vi "FisherPaykel Set Agitate Profile.vi"(0 "VISA Refnum in":refnum<visa-resource-name>, 1 "Agitate Parameters":T2 {"PauseTime (0-1800ms 10ms Increment)" step=10; "PlateauTime (0-1800ms 10ms Increment)" step=10; "TargetSpeed (0-200RPM)" max=1600 step=1; "RampUpTime (1-600ms)" max=600 step=10; "Agitate Running Time (sec)" step=1}, 2 "GEA2 Reference In":refnum<k24>, 5 "Error In":errorcluster, 7 "Main Command":T4=">PA", 8 "Debug":bool, 10 "Use GEA Inverter Output":bool, 13 "GEA Inputs":T1={"Source"=228, "Destination"=35} {"Destination" format="%.0x"; "Source" format="%.0x"}) -> (14 "VISA resource name out":refnum<visa-resource-name>, 15 "Agitate Parameters Out":T2 {"PauseTime (0-1800ms 10ms Increment)" step=10; "PlateauTime (0-1800ms 10ms Increment)" step=10; "TargetSpeed (0-200RPM)" max=1600 step=1; "RampUpTime (1-600ms)" max=600 step=10; "Agitate Running Time (sec)" step=1}, 16 "GEA2 Reference Out":refnum<k24>, 19 "Error Out":errorcluster)   [LabVIEW 2016]
uses:
  Type Definitions/Fisher Paykel Main Command.ctl
  Type Definitions/Fisher Paykel Agitate Parameters.ctl
  Type Definitions/FisherPaykel Direction CMD.ctl
  Trunk/Utility/LabVIEW GEA2 Toolkit v1.0.0.0/type defs/Source_Destination.ctl
  C:/Technology Lab/NI-2010/Trunk/Utility/LabVIEW GEA2 Toolkit v1.0.0.0/Appliance.NET/GeaCommunication.dll
  Trunk/Utility/LabVIEW GEA2 Toolkit v1.0.0.0/Appliance.NET/GeaCommunication.dll
  Trunk/Utility/LabVIEW GEA2 Toolkit v1.0.0.0/type defs/ERD Write Data In.ctl
  Trunk/Utility/LabVIEW GEA2 Toolkit v1.0.0.0/type defs/Data Type.ctl
  Trunk/Utility/LabVIEW GEA2 Toolkit v1.0.0.0/library/GEA2_Toolkit.lvlib
panel:
  out "Command (Debug)":string
  # "Agitate Profile Parameters"
  # "Agitate Start Parameters"
  # "Agitate Profile Parameters"
  # "Agitate Start Parameters"
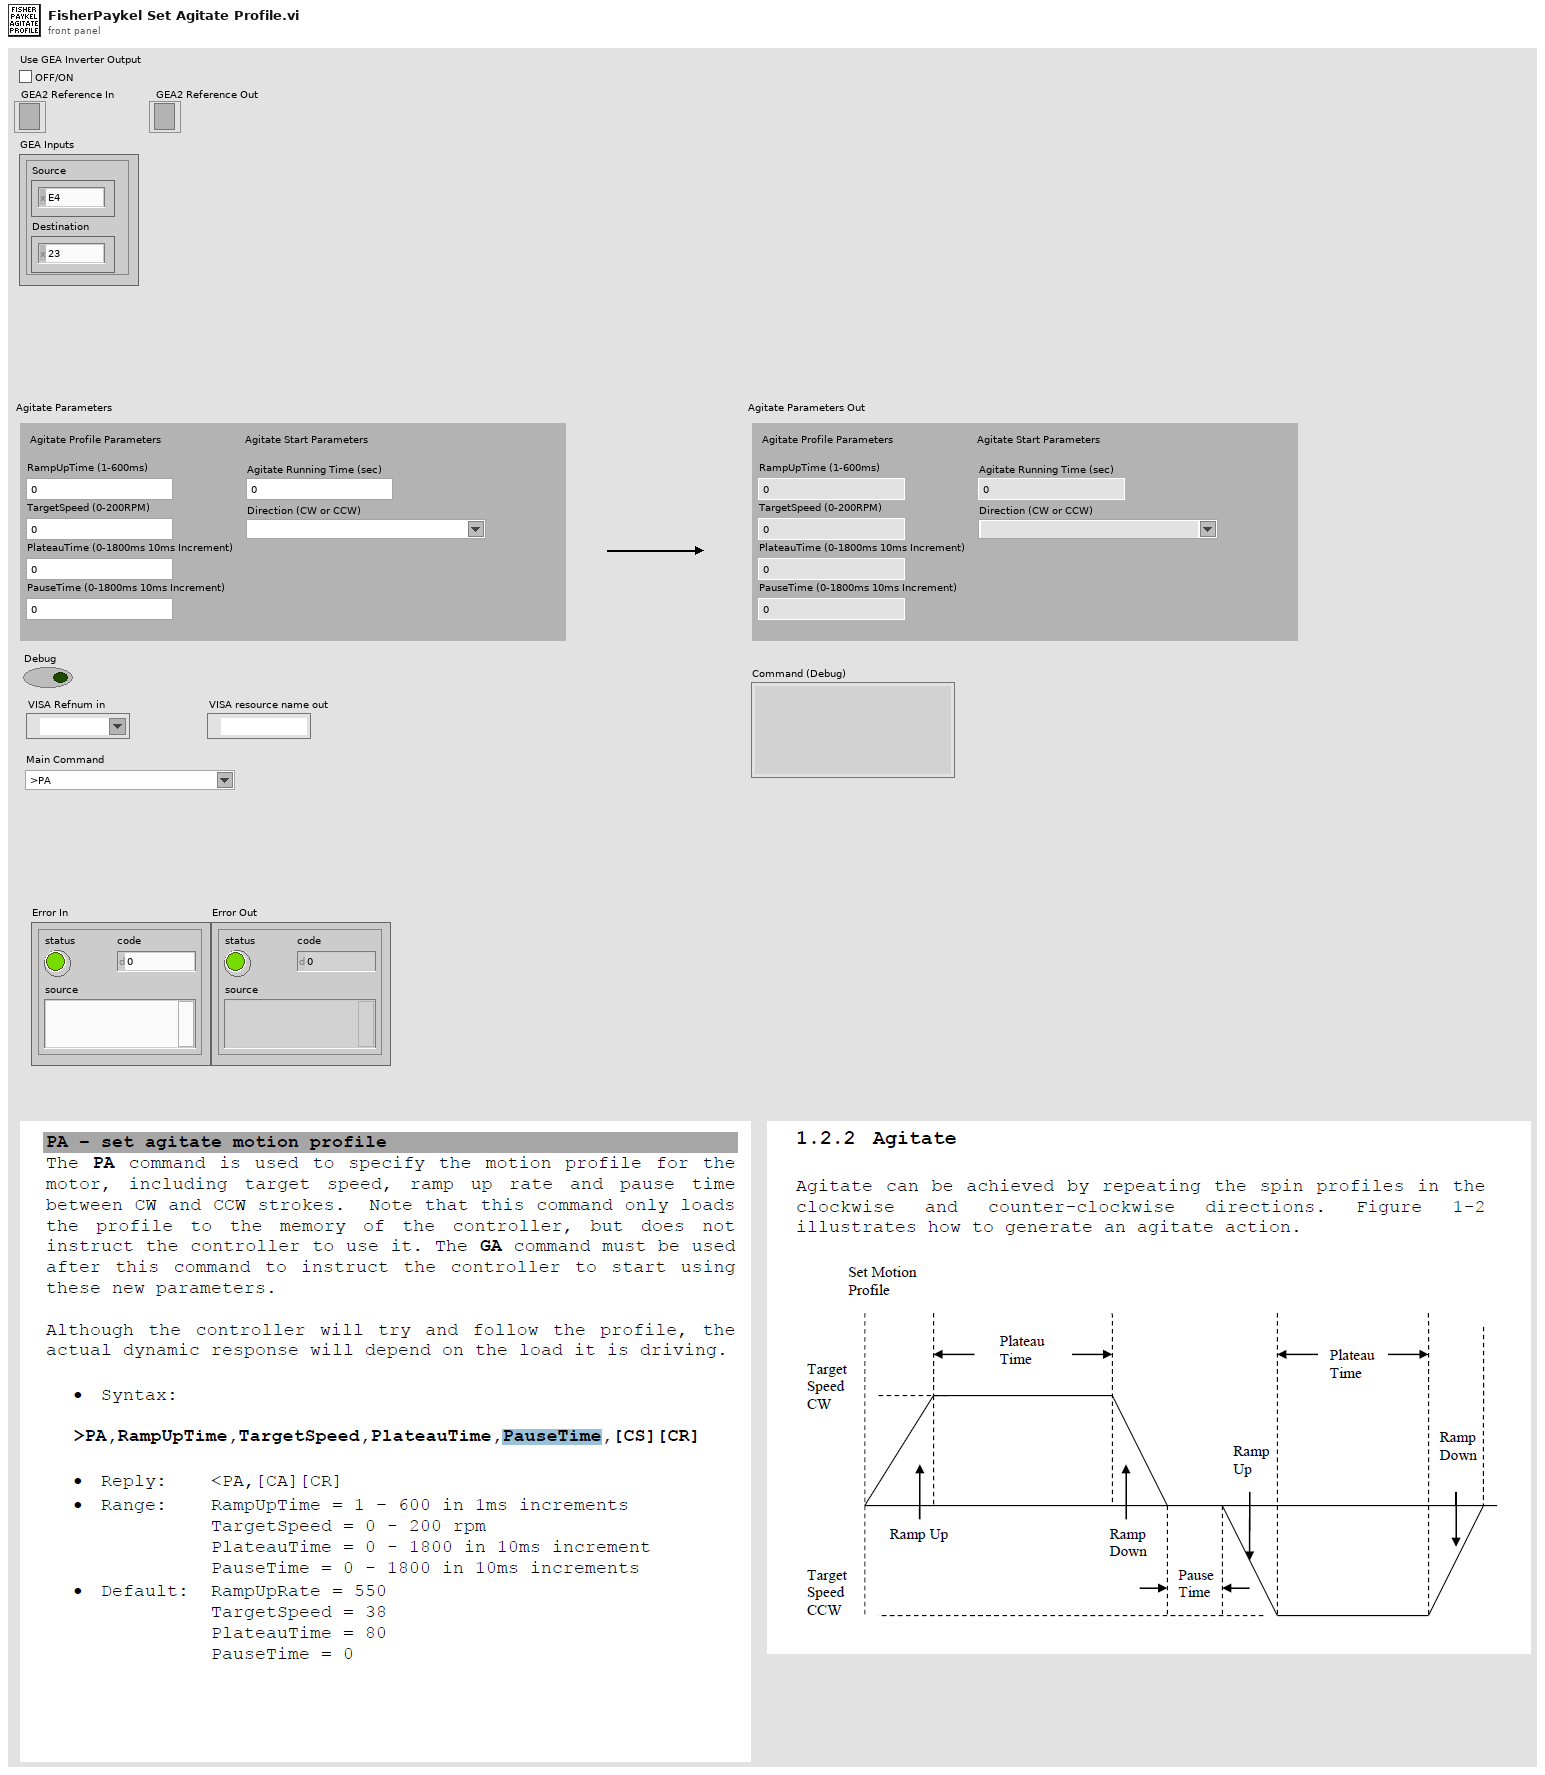
[diagram p1: front panel]
types:
  T1 = typedef "GEA2_Toolkit.lvlib/Source_Destination.ctl" = cluster{"Source":u8, "Destination":u8}
  T2 = typedef "Fisher Paykel Agitate Parameters.ctl" = cluster{"Agitate Running Time (sec)":u16, "Direction (CW or CCW)":T3, "RampUpTime (1-600ms)":u16, "TargetSpeed (0-200RPM)":u16, "PlateauTime (0-1800ms 10ms Increment)":u16, "PauseTime (0-1800ms 10ms Increment)":u16}
  T3 = typedef "FisherPaykel Direction CMD.ctl" = string
  T4 = typedef "Fisher Paykel Main Command.ctl" = string
  T5 = typedef "GEA2_Toolkit.lvlib/ERD Write Data In.ctl" = cluster{"ERD Number":u16, "Data Type":T6, "Data":string}
  T6 = typedef "GEA2_Toolkit.lvlib/Data Type.ctl" = enum16{"string", "boolean", "uint8_t", "uint16_t", "uint32_t", "uint64_t"}
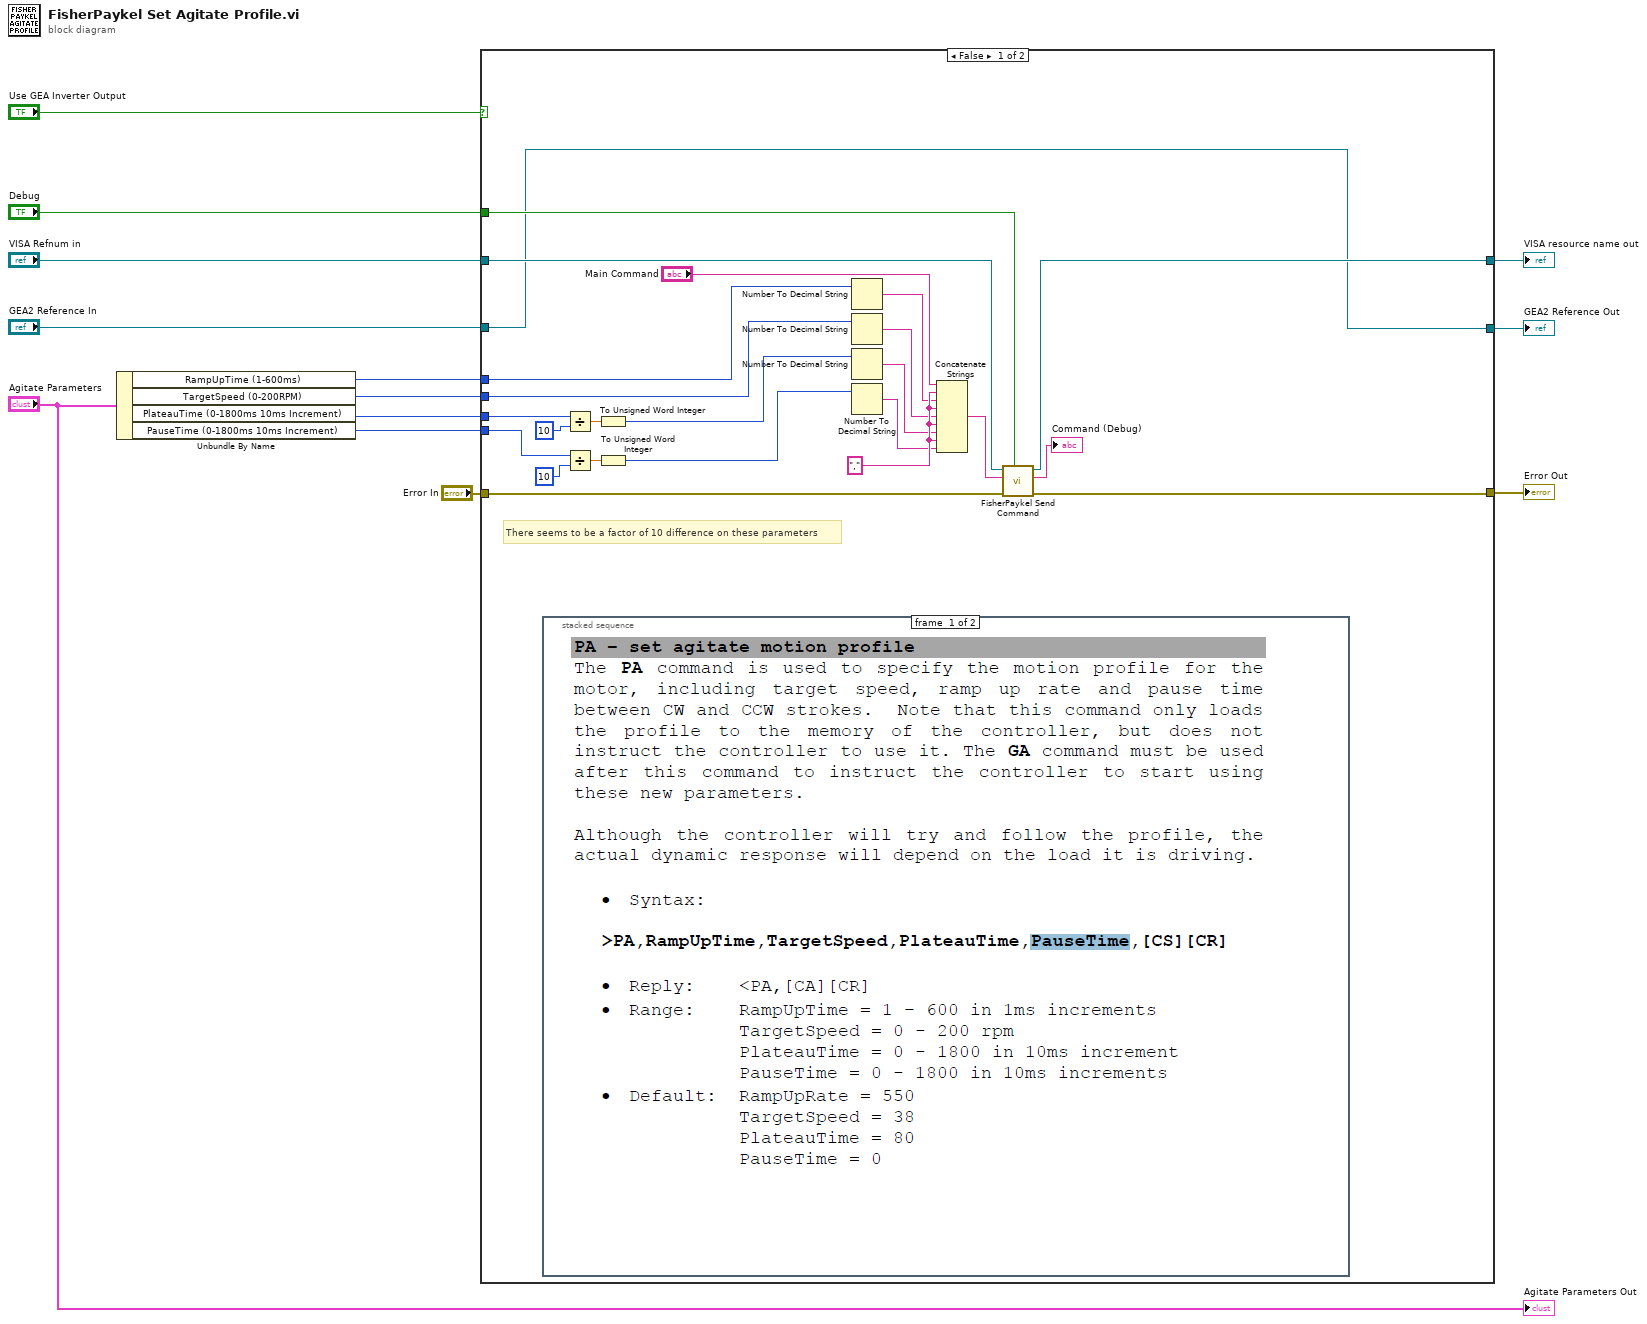
[diagram p0: block diagram]
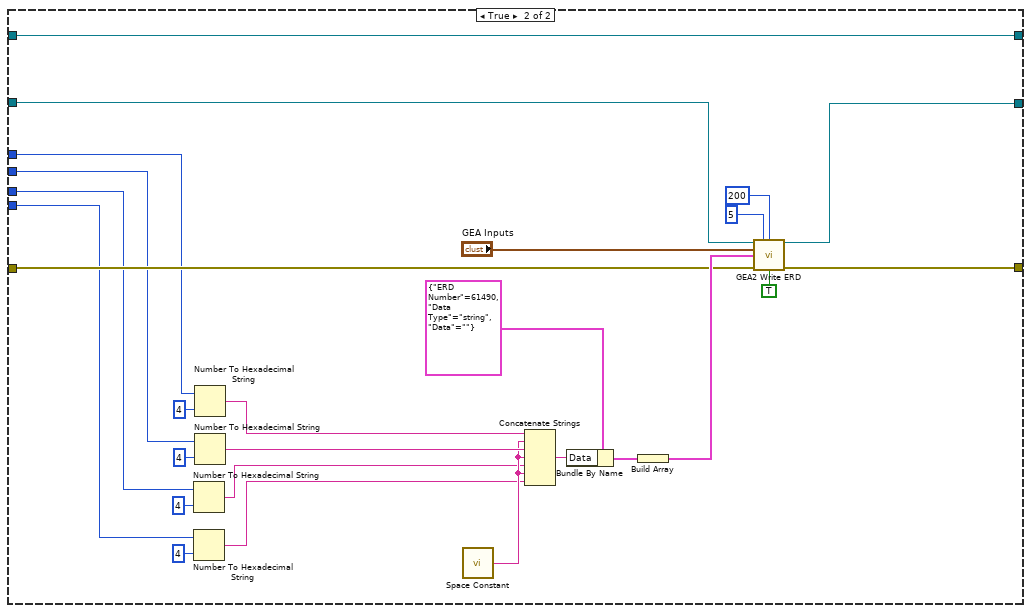
[diagram p3: hidden frame]
diagram:
  n1 = Unbundle By Name("Agitate Parameters") -> ("RampUpTime (1-600ms)"=w9:u16, "TargetSpeed (0-200RPM)"=w8:u16, "PlateauTime (0-1800ms 10ms Increment)"=w2:u16, "PauseTime (0-1800ms 10ms Increment)"=w1:u16)
  n2 = case shown="False" "Use GEA Inverter Output" {
    tunnel: [w37 w50] -> w13
    tunnel: "VISA Refnum in" -> [w36 w63]
    tunnel: "Debug" -> [w35 _]
    tunnel: w9 -> [w30 w43]
    tunnel: w8 -> [w29 w42]
    tunnel: w2 -> [w19 w41]
    tunnel: w1 -> [w15 w40]
    tunnel: [w24 w63] -> w6
    tunnel: "Error In" -> [w23 w49]
    tunnel: "GEA2 Reference In" -> [w22 w48]
    tunnel: [w22 w47] -> w3
    frame False {
      w33 = ","
      # "There seems to be a factor of 10 difference on these parameters"
      n3 = stacked-sequence {
        frame #0 {
        }
        frame #1 {
        }
      }
      n4 = Divide(x=w19, y=u16 10) -> (x/y=w21:dbl)
      n5 = Divide(x=w15, y=u16 10) -> (x/y=w17:dbl)
      n6 = To Unsigned Word Integer(number=w21) -> (unsigned 16bit integer=w18:u16)
      n7 = To Unsigned Word Integer(number=w17) -> (unsigned 16bit integer=w14:u16)
      n8 = Number To Decimal String(number=w30) -> (decimal integer string=w28:string)  [unwired: 1 in]
      n9 = Number To Decimal String(number=w29) -> (decimal integer string=w27:string)  [unwired: 1 in]
      n10 = Number To Decimal String(number=w18) -> (decimal integer string=w26:string)  [unwired: 1 in]
      n11 = Number To Decimal String(number=w14) -> (decimal integer string=w25:string)  [unwired: 1 in]
      n12 = Concatenate Strings("Main Command", w33, w28, w33, w27, w33, w26, w33, w25) -> (w32:string)
      n13 = call "FisherPaykel Send Command.vi"("Debug"=w35, "error in (no error)"=w23, "Send Command"=w32, "VISA Refnum in"=w36) -> ("error out"=w37:errorcluster, "Command (Debug)"=→"Command (Debug)":string, "VISA Refnum out"=w24:refnum<visa-resource-name>)  [unwired: 5 in]
    }
    frame True {
      n14 = Number To Hexadecimal String(1:i16 4 ("width (-)"), 2:w41) -> (0:w39:string)
      n15 = Number To Hexadecimal String(1:i16 4 ("width (-)"), 2:w40) -> (0:w38:string)
      n16 = Number To Hexadecimal String(1:i16 4 ("width (-)"), 2:w43) -> (0:w55:string)
      n17 = Number To Hexadecimal String(1:i16 4 ("width (-)"), 2:w42) -> (0:w56:string)
      n18 = call <vilib>:"Space Constant.vi"() -> ("String"=w46:string)
      n19 = Concatenate Strings(w55, w46, w56, w46, w39, w46, w38) -> (w59:string)
      n20 = Bundle By Name(cluster=T5 {"ERD Number"=61490, "Data Type"=enum."string", "Data"=""} ("ERD Write Data In"), "Data"=w59) -> (w60:T5)
      n21 = Build Array(w60) -> (w57:T5[])
      n22 = call "GEA2 Write ERD.vi"("GEA2 Reference In"=w48, "Retry Count"=5, "Read Timeout (ms)"=u32 200, "GEA Inputs"="GEA Inputs", "Write ERD List"=w57, "Error In"=w49, "Verify ERD Response?"=TRUE) -> ("GEA2 Reference Out"=w47:refnum<k24>, "Error Out"=w50:errorcluster)  [unwired: 6 in, 1 out]
    }
  }
  "Error Out" <- w13
  "VISA resource name out" <- w6
  "GEA2 Reference Out" <- w3
  "Agitate Parameters Out" <- "Agitate Parameters"
